vi "Set IO Out State.vi"(10 "state":u8, 11 "channel":u8) -> ()   [LabVIEW 2021, in "vmmso.lvlib"]
doc: "DLL_API void WINAPI SetIOOutState(unsigned char channel, unsigned char state);"
uses:
  vmmso.lvlib
  vmmso.dll
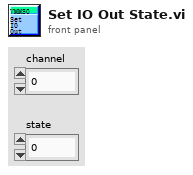
[diagram p1: front panel]
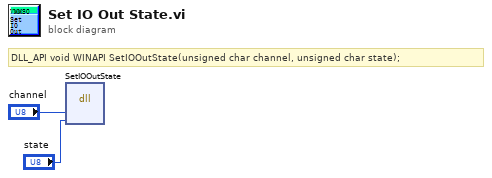
[diagram p0: block diagram]
diagram:
  # "DLL_API void WINAPI SetIOOutState(unsigned char channel, unsigned char state);"
  n1 = dll-call lib="D:/labviewdemo/LabviewDemo 21/vmmso/vmmso.*" fn="SetIOOutState"("channel"="channel", "state"="state") -> ()  [unwired: 6 in, 2 out]
